vi "isPathNotHidden.vi"(11 "pathIn":path) -> (1 "pathNotHidden":bool, 2 "pathIsHidden":bool, 3 "pathOut":path)   [LabVIEW 2020]
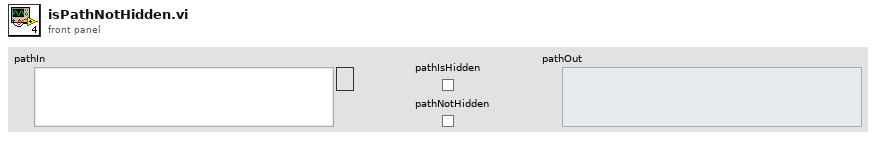
[diagram p1: front panel]
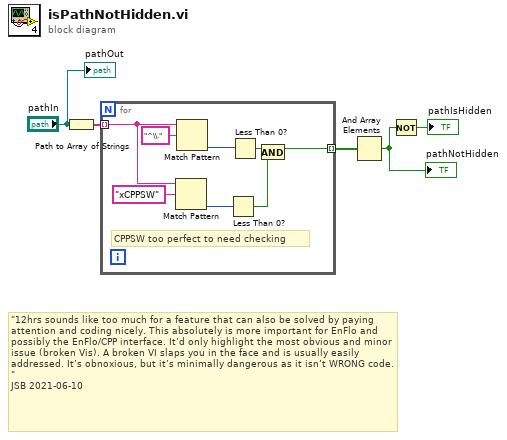
[diagram p0: block diagram]
diagram:
  # "\"12hrs sounds like too much for a feature that can also be solved by paying attention and coding nicely. This absolutely is more important for EnFlo and possibly the EnFlo/CPP interface. It’d only highlight the most obvious and minor issue (broken Vis). A broken VI slaps you in the face and is usually easily addressed. It’s obnoxious, but it’s minimally dangerous as it isn’t WRONG code.\"\nJSB 2021-06-10"
  n1 = Path to Array of Strings(0:"pathIn") -> (2:w5:string[])  [unwired: 1 out]
  n2 = for {
    tunnel: w5 -> [w9] mode=indexing
    tunnel: [w7] -> w3 mode=indexing
    # "CPPSW too perfect to need checking"
    n3 = Match Pattern(string=w9, regular expression="xCPPSW") -> (offset past match=w8:i32)  [unwired: 1 in, 3 out]
    n4 = Match Pattern(string=w9, regular expression="^\\.") -> (offset past match=w12:i32)  [unwired: 1 in, 3 out]
    n5 = Less Than 0?(x=w8) -> (x < 0?=w6:bool)
    n6 = Less Than 0?(x=w12) -> (x < 0?=w11:bool)
    n7 = And(x=w11, y=w6) -> (x .and. y?=w7:bool)
  }
  n8 = And Array Elements(Boolean array=w3) -> (logical AND=w2:bool)
  "pathNotHidden" <- w2
  n9 = Not(x=w2) -> (.not. x?=→"pathIsHidden":bool)
  "pathOut" <- "pathIn"
